vi "Get DQMH Main VI.vi"(8 "error in (no error)":errorcluster, 11 "Library Ref in":refnum<vi>) -> (0 "error out":errorcluster, 2 "Main VI Ref":refnum<vi>, 3 "Library Ref out":refnum<vi>)   [LabVIEW 2017, in "Open DQMH Request Message Diagram.lvlib"]
doc: "Returns the Main VI of the DQMH Module of the selected SubVI.\n\nBSD 3-Clause License\n\nCopyright (c) 2022, Neosoft Technologies Inc\nAll rights reserved.\n\nRedistribution and use in source and binary forms, with or without\nmodification, are permitted provided that the following conditions are met:\n\n1. Redistributions of source code must retain the above copyright notice, this\n list of conditions and the following disclaimer.\n\n2. Redistributions in binary form must reproduce the above copyright notice,\n this list of conditions and the following disclaimer in the documentation\n and/or other materials provided with the distribution.\n\n3. Neither the name of the copyright holder nor the names of its\n contributors may be used to endorse or promote products derived from\n this software without specific prior written permission.\n\nTHIS SOFTWARE IS PROVIDED BY THE COPYRIGHT HOLDERS AND CONTRIBUTORS \"AS IS\"\nAND ANY EXPRESS OR IMPLIED WARRANTIES, INCLUDING, BUT NOT LIMITED TO, THE\nIMPLIED WARRANTIES OF MERCHANTABILITY AND FITNESS FOR A PARTICULAR PURPOSE ARE\nDISCLAIMED. IN NO EVENT SHALL THE COPYRIGHT HOLDER OR CONTRIBUTORS BE LIABLE\nFOR ANY DIRECT, INDIRECT, INCIDENTAL, SPECIAL, EXEMPLARY, OR CONSEQUENTIAL\nDAMAGES (INCLUDING, BUT NOT LIMITED TO, PROCUREMENT OF SUBSTITUTE GOODS OR\nSERVICES; LOSS OF USE, DATA, OR PROFITS; OR BUSINESS INTERRUPTION) HOWEVER\nCAUSED AND ON ANY THEORY OF LIABILITY, WHETHER IN CONTRACT, STRICT LIABILITY,\nOR TORT (INCLUDING NEGLIGENCE OR OTHERWISE) ARISING IN ANY WAY OUT OF THE USE\nOF THIS SOFTWARE, EVEN IF ADVISED OF THE POSSIBILITY OF SUCH DAMAGE."
uses:
  Open DQMH Request Message Diagram.lvlib
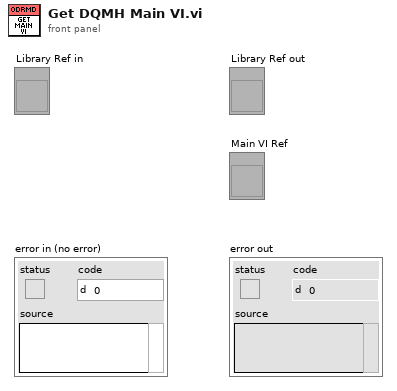
[diagram p1: front panel]
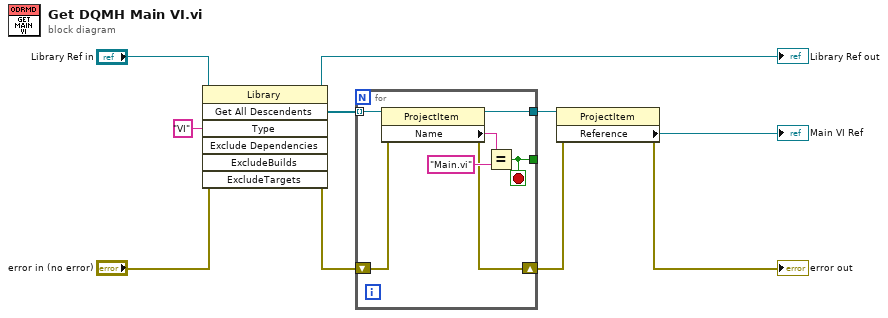
[diagram p0: block diagram]
diagram:
  n1 = invoke class="Library" method="Get All Descendents"(reference="Library Ref in", error in="error in (no error)", "Type"="VI") -> (reference out=→"Library Ref out":refnum<vi>, error out=w6:errorcluster, "All Descendents"=w3:refnum<vi>[])  [unwired: 4 in, 4 out]
  n2 = for {
    tunnel: w3 -> [w17] mode=indexing
    tunnel: [w11] -> _
    tunnel: [w14] -> w4
    shift-right: [w12] -> w7
    shift-left: w6 -> [w13]
    stop <- w11 stop-if-true
    n3 = property class="ProjectItem"(reference=w17, error in=w13) -> (reference out=w14:refnum<vi>, error out=w12:errorcluster, "Name"=w16:string)
    n4 = Equal?(x=w16, y="Main.vi") -> (x = y?=w11:bool)
  }
  n5 = property class="ProjectItem"(reference=w4, error in=w7) -> (error out=→"error out":errorcluster, "Reference"=→"Main VI Ref":refnum<vi>)  [unwired: 1 out]
